vi "svacg_Create Log Scale Linear Interpolated Specifications.vi"(6 "Log Specs":bool, 8 "error in (no error)":errorcluster, 9 "x0":dbl=100.0 format="%.2f", 10 "dx":dbl=100.0 format="%.2f", 11 "raw specifications":cluster{"X-specs":dbl[], "Y-specs":dbl[]} {"Y-specs" format="%.2p"; "X-specs" format="%.2p"}) -> (0 "error out":errorcluster, 1 "x0 out":dbl=100.0 format="%.2f", 2 "dx out":dbl=100.0 format="%.2f", 3 "XY pairs output":cluster{"X-data":dbl[], "Y-data":dbl[]} {"Y-data" format="%0.2f"; "X-data" format="%0.2f"})   [LabVIEW 2017]
panel:
  out "x0-dt-Y output":cluster{"x0":dbl, "dX":dbl, "Y-data":dbl[]} {"Y-data" format="%0.2f"; "dX" format="%0.2f"; "x0" format="%0.2f"}
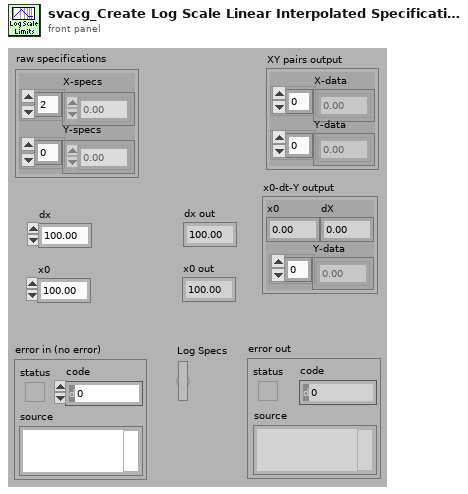
[diagram p1: front panel]
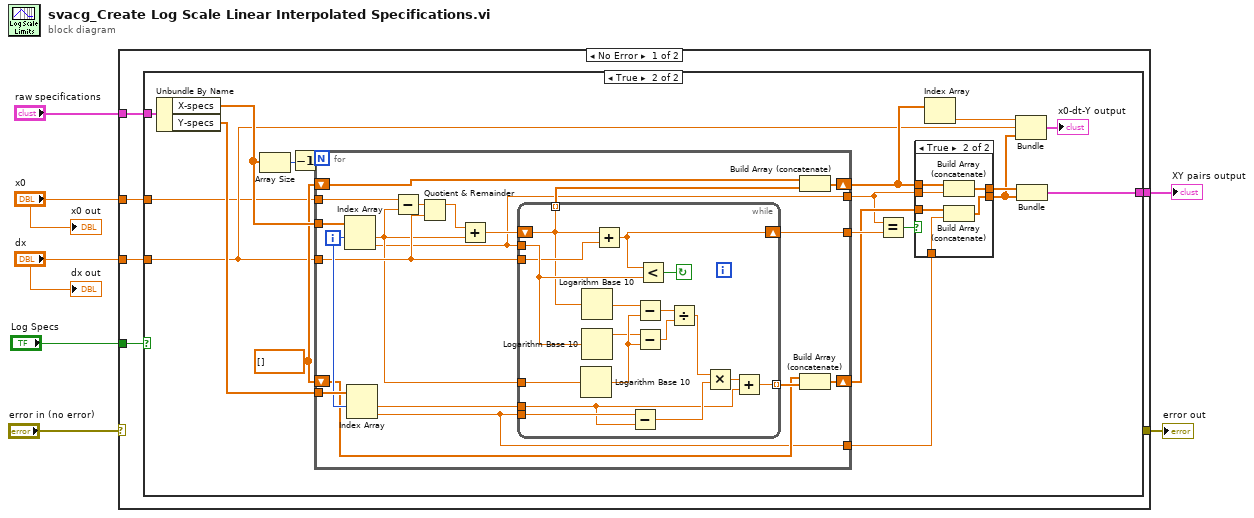
[diagram p0: block diagram]
diagram:
  n1 = case shown="No Error" "error in (no error)" {
    selector: "error in (no error)" -> [_ w77]
    tunnel: [w12 _] -> w7
    tunnel: "raw specifications" -> [w11 _]
    tunnel: "dx" -> [w10 _]
    tunnel: "x0" -> [w9 _]
    tunnel: "Log Specs" -> [w8 _]
    tunnel: [_ w77] -> w1
    frame No Error {
      n2 = case shown="True" w8 {
        tunnel: [w13 w32] -> w12
        tunnel: w11 -> [w13 w29]
        tunnel: w10 -> [_ w15]
        tunnel: w9 -> [_ w14]
        frame False {
        }
        frame True {
          w24 = dbl[] []
          n3 = Unbundle By Name(w29) -> ("X-specs"=w27:dbl[], "Y-specs"=w28:dbl[])
          n4 = Array Size(array=w27) -> (size(s)=w26:i32)
          n5 = Decrement(x=w26) -> (x-1=w25:i32)
          n6 = for {
            N: w25 -> [_]
            tunnel: w27 -> [w59]
            tunnel: w28 -> [w58]
            shift-right: [w53] -> w19
            shift-left: w24 -> [w54]
            tunnel: w15 -> [w48]
            shift-right: [w50] -> w21
            shift-left: w24 -> [w51]
            tunnel: w14 -> [w44]
            tunnel: [w43] -> w23
            tunnel: [w42] -> w17
            tunnel: [w41] -> w16
            i -> [w57]
            n7 = Index Array(array=w59, index #1=w57) -> (element #1=w45:dbl, element #2=w42:dbl)  [unwired: 1 in]
            n8 = Index Array(array=w58, index #1=w57) -> (element #1=w56:dbl, element #2=w41:dbl)  [unwired: 1 in]
            n9 = Subtract(x=w44, y=w45) -> (x-y=w49:dbl)
            n10 = Quotient & Remainder(x=w49, y=w48) -> (x-y*floor(x/y)=w47:dbl)  [unwired: 1 out]
            n11 = Add(x=w47, y=w45) -> (x+y=w46:dbl)
            n12 = while {
              tunnel: w42 -> [w76]
              shift-right: [w64] -> w43
              shift-left: w46 -> [w63]
              tunnel: w45 -> [w75]
              tunnel: w41 -> [w71]
              tunnel: w56 -> [w60]
              tunnel: [w67] -> w55 mode=indexing
              tunnel: w48 -> [w66]
              tunnel: [w63] -> w52 mode=indexing
              stop <- w65 continue-if-true
              n13 = Logarithm Base 10(1:w75) -> (0:w73:dbl)
              n14 = Logarithm Base 10(1:w63) -> (0:w62:dbl)
              n15 = Logarithm Base 10(1:w76) -> (0:w61:dbl)
              n16 = Add(x=w63, y=w66) -> (x+y=w64:dbl)
              n17 = Subtract(x=w71, y=w60) -> (x-y=w69:dbl)
              n18 = Subtract(x=w62, y=w73) -> (x-y=w74:dbl)
              n19 = Subtract(x=w61, y=w73) -> (x-y=w72:dbl)
              n20 = Less?(x=w64, y=w76) -> (x < y?=w65:bool)
              n21 = Divide(x=w74, y=w72) -> (x/y=w70:dbl)
              n22 = Multiply(x=w70, y=w69) -> (x*y=w68:dbl)
              n23 = Add(x=w68, y=w60) -> (x+y=w67:dbl)
            }
            n24 = Build Array (concatenate)(w51, w52) -> (w50:dbl[])
            n25 = Build Array (concatenate)(w54, w55) -> (w53:dbl[])
          }
          n26 = Equal?(x=w17, y=w23) -> (x = y?=w22:bool)
          n27 = case shown="True" w22 {
            tunnel: [w34 w40] -> w20
            tunnel: w21 -> [w34 w39]
            tunnel: w19 -> [w33 w37]
            tunnel: [w33 w38] -> w18
            tunnel: w17 -> [_ w36]
            tunnel: w16 -> [_ w35]
            frame False {
            }
            frame True {
              n28 = Build Array (concatenate)(w39, w36) -> (w40:dbl[])
              n29 = Build Array (concatenate)(w37, w35) -> (w38:dbl[])
            }
          }
          n30 = Index Array(array=w21) -> (element=w31:dbl)  [unwired: 1 in]
          n31 = Bundle(w31, "dx"=w15, w18) -> (→"x0-dt-Y output":cluster{dbl, "dx":dbl, dbl[]})  [unwired: 1 in]
          n32 = Bundle(w20, w18) -> (w32:cluster{dbl[], dbl[]})  [unwired: 1 in]
        }
      }
    }
    frame Error {
    }
  }
  "XY pairs output" <- w7
  "error out" <- w1
  "dx out" <- "dx"
  "x0 out" <- "x0"
